vi "Create Virtual Axis (by Angle).vi"(6 "Axis Numbers (1,2)":i32[](array[numeric])=[1, 2], 7 "Angle":dbl min=-360.0 max=360.0 step=0.1 format="%#.1f", 8 "error in (no error)":errorcluster, 9 "Device Number":string, 10 "Virtual Axis Number (1)":i32=1, 11 "VISA resource name":refnum<visa-resource-name>) -> (0 "error out":errorcluster, 3 "VISA resource name out":refnum<visa-resource-name>)   [LabVIEW 2015, in "Zaber A Series.lvlib"]
doc: "Configured a virtual axis on a device that supports it. A virtual axis defines an angular relationship between two axes such that when the virtual axis is moved, both axes move in proportion to the angle. Normal single-axis move commands can still be used while a virtual axis is configured, but will only move one axis at a time.\n\nTo configure a virtual axis you must specify an identifying number for it, between 1 and the value of the \"virtual.numvirtual\" device setting. You must also specify two axis numbers to be members of the group, and the angle in degrees (with one decimal point of precision) of the second axis relative to the first.\n\nTo use the features of a virtual axis you must use the virtual axis specific VIs provided.\n\nThis VI does not check in advance for error conditions such as lockstep not being supported on the device or no virtual axis numbers being available.\n\nThis VI requires that the Initialize VI has been called with the same serial port."
uses:
  Zaber A Series.lvlib
  Private/All Commands.ctl
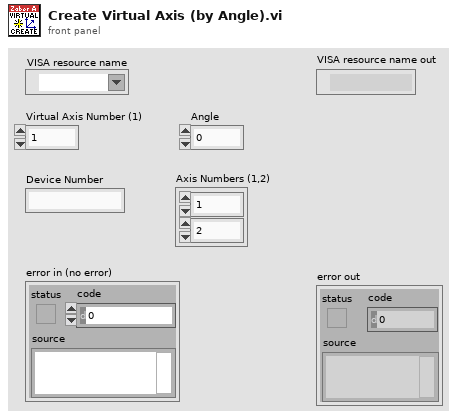
[diagram p1: front panel]
types:
  T1 = typedef "Zaber A Series.lvlib/All Commands.ctl" = string
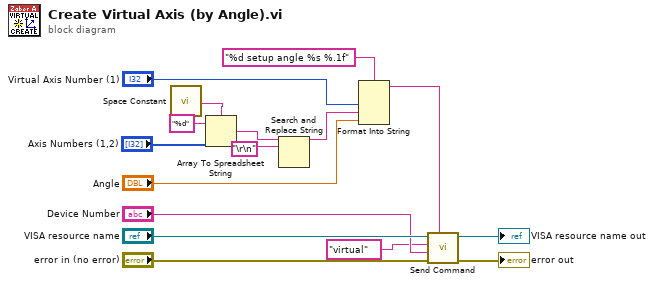
[diagram p0: block diagram]
diagram:
  n1 = call <vilib>:"Space Constant.vi"() -> ("String"=w12:string)
  n2 = Array To Spreadsheet String(delimiter (Tab)=w12, array="Axis Numbers (1,2)", 3:"%d" ("format string")) -> (spreadsheet string=w13:string)
  n3 = Search and Replace String(input string=w13, search string="\r\n") -> (result string=w5:string)  [unwired: 6 in, 3 out]
  n4 = Format Into String(format string="%d setup angle %s %.1f", "Virtual Axis Number (1)", w5, "Angle") -> (resulting string=w3:string)  [unwired: 2 in, 1 out]
  n5 = call "Send Command.vi"("Data"=w3, "error in (no error)"="error in (no error)", "Device and Axis"="Device Number", "Command"=T1 "virtual" ("Complete Command List"), "VISA resource name"="VISA resource name") -> ("error out"=→"error out":errorcluster, "VISA resource name out"=→"VISA resource name out":refnum<visa-resource-name>)  [unwired: 1 in, 4 out]
